vi "Scaling-wall-pos.vi"(8 "error in (no error)":errorcluster, 10 "Interpolation Points":dbl[][](array[numeric])=[[0.0, 15.0], [1.0, 30.0]], 11 "Input":dbl=1.0 caption="m") -> (0 "error out":errorcluster, 3 "Output":dbl)   [LabVIEW 2018]
doc: "Changes the amplitude of a signal by scaling or mapping the signal.\n--------------------\n\nThis Express VI is configured as follows:\n\nScaling Type: Interpolated"
uses:
  <vilib>/express/express shared/scalingTypes.ctl
panel:
  in  "Lowest Peak":dbl
  in  "Highest Peak":dbl=1.0
  in  "dB Reference":dbl=1.0
  in  "m":dbl=1.0
  in  "b":dbl
  in  "Scaling Type":T1=enum."Interpolation"
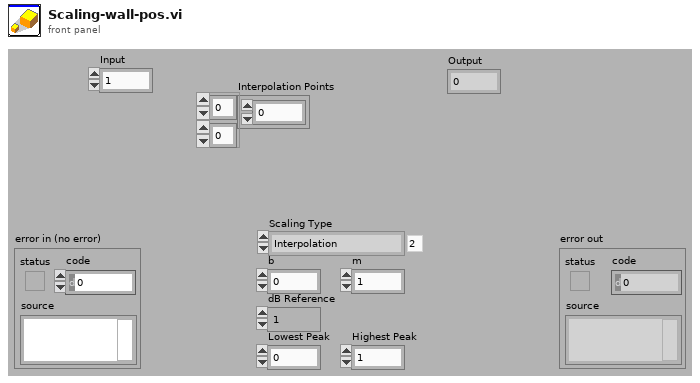
[diagram p1: front panel]
types:
  T1 = typedef "scalingTypes.ctl" = enum16{"Normalize", "Linear", "Interpolation", "Logarithmic"}
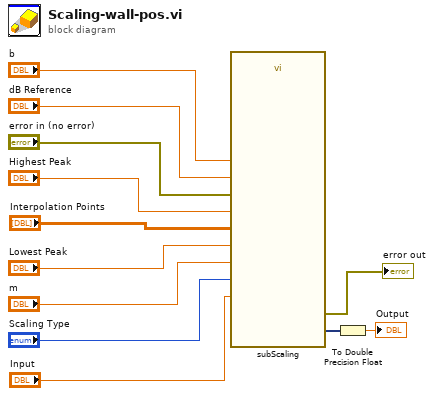
[diagram p0: block diagram]
diagram:
  n1 = call <vilib>:"subScaling.vi"("Signals"="Input", "b"="b", "m"="m", "dB reference"="dB Reference", "Scaling Type"="Scaling Type", "error in (no error)"="error in (no error)", "Interpolation Points"="Interpolation Points", "Highest Peak"="Highest Peak", "Lowest Peak"="Lowest Peak") -> ("Scaled Signals"=w3:dynamicdata, "error out"=→"error out":errorcluster)  [unwired: 5 in]
  n2 = To Double Precision Float(number=w3) -> (double precision float=→"Output":dbl)
